vi "TrapezoidalMotionProfile.vi"(8 "dt":u32=20, 11 "Config":T1={"Distance"=200.0, "MaxVelocity"=100.0, "MaxAccel"=75.0, "InitialVelocity"=0.0, "FinalVelocity"=0.0}) -> (0 "dt":u32=20, 3 "Profile":cluster{"Pos":dbl, "Vel":dbl, "Accel":dbl}[](array[cluster]))   [LabVIEW 2016]
panel:
  out "Graph":dbl[][](graph)=[[0.0, 0.015000000000000001, 0.060000000000000005, 0.135, 0.24000000000000002, 0.37500000000000006, 0.54, 0.7350000000000001, 0.9600000000000001, 1.2149999999999999, 1.5000000000000002, 1.815, 2.16, 2.535, 2.9400000000000004, 3.375, 3.8400000000000003, 4.335000000000001, 4.859999999999999, 5.415, 6.000000000000001, 6.614999999999999, 7.26, 7.9350000000000005, 8.64, 9.375, 10.14, 10.935, 11.760000000000002, 12.614999999999998, 13.5, 14.415000000000001, 15.360000000000001, 16.335, 17.340000000000003, 18.375000000000004, 19.439999999999998, 20.535, 21.66, 22.815, 24.000000000000004, 25.215000000000003, 26.459999999999997, 27.734999999999996, 29.04, 30.375000000000004, 31.740000000000002, 33.135000000000005, 34.56, 36.015, 37.5, 39.015, 40.56, 42.135000000000005, 43.74, 45.37500000000001, 47.040000000000006, 48.735000000000014, 50.459999999999994, 52.214999999999996, 54.0, 55.815, 57.660000000000004, 59.535000000000004, 61.440000000000005, 63.37500000000001, 65.34, 67.33333333333334, 69.33333333333334, 71.33333333333334, 73.33333333333334, 75.33333333333333, 77.33333333333333, 79.33333333333333, 81.33333333333333, 83.33333333333333, 85.33333333333333, 87.33333333333334, 89.33333333333334, 91.33333333333334, 93.33333333333334, 95.33333333333334, 97.33333333333334, 99.33333333333334, 101.33333333333333, 103.33333333333333, 105.33333333333333, 107.33333333333333, 109.33333333333333, 111.33333333333334, 113.33333333333334, 115.33333333333334, 117.33333333333334, 119.33333333333334, 121.33333333333334, 123.33333333333334, 125.33333333333331, 127.33333333333333, 129.33333333333331, 131.33333333333331, 133.33333333333331, 135.31833333333338, 137.27333333333337, 139.19833333333338, 141.09333333333336, 142.95833333333337, 144.79333333333338, 146.59833333333336, 148.37333333333336, 150.11833333333337, 151.83333333333337, 153.51833333333337, 155.17333333333337, 156.79833333333337, 158.39333333333337, 159.95833333333337, 161.49333333333334, 162.99833333333333, 164.47333333333336, 165.91833333333335, 167.33333333333334, 168.71833333333336, 170.07333333333335, 171.39833333333334, 172.69333333333336, 173.95833333333334, 175.19333333333336, 176.39833333333337, 177.57333333333335, 178.71833333333336, 179.83333333333334, 180.91833333333335, 181.97333333333336, 182.99833333333336, 183.99333333333337, 184.95833333333334, 185.89333333333335, 186.79833333333335, 187.67333333333335, 188.51833333333335, 189.33333333333334, 190.11833333333334, 190.87333333333333, 191.59833333333333, 192.29333333333335, 192.95833333333334, 193.59333333333333, 194.19833333333335, 194.77333333333334, 195.31833333333333, 195.83333333333334, 196.31833333333333, 196.77333333333334, 197.19833333333335, 197.59333333333333, 197.95833333333334, 198.29333333333335, 198.59833333333333, 198.87333333333333, 199.11833333333334, 199.33333333333334, 199.51833333333335, 199.67333333333335, 199.79833333333335, 199.89333333333335, 199.95833333333334, 199.99333333333334, 199.99833333333333], [0.0, 1.5, 3.0, 4.5, 6.0, 7.5, 9.0, 10.500000000000002, 12.0, 13.5, 15.0, 16.5, 18.0, 19.5, 21.000000000000004, 22.5, 24.0, 25.500000000000004, 27.0, 28.5, 30.0, 31.5, 33.0, 34.5, 36.0, 37.5, 39.0, 40.5, 42.00000000000001, 43.5, 45.0, 46.5, 48.0, 49.5, 51.00000000000001, 52.50000000000001, 54.0, 55.5, 57.0, 58.5, 60.0, 61.50000000000001, 63.0, 64.5, 66.0, 67.5, 69.0, 70.5, 72.0, 73.5, 75.0, 76.5, 78.0, 79.5, 81.0, 82.5, 84.00000000000001, 85.50000000000001, 87.0, 88.5, 90.0, 91.5, 93.0, 94.5, 96.0, 97.5, 99.0, 100.0, 100.0, 100.0, 100.0, 100.0, 100.0, 100.0, 100.0, 100.0, 100.0, 100.0, 100.0, 100.0, 100.0, 100.0, 100.0, 100.0, 100.0, 100.0, 100.0, 100.0, 100.0, 100.0, 100.0, 100.0, 100.0, 100.0, 100.0, 100.0, 100.0, 100.0, 100.0, 100.0, 100.0, 98.5, 97.0, 95.5, 94.0, 92.5, 91.0, 89.49999999999999, 87.99999999999999, 86.49999999999999, 84.99999999999999, 83.49999999999999, 81.99999999999999, 80.49999999999999, 78.99999999999999, 77.49999999999997, 76.00000000000001, 74.50000000000001, 73.00000000000001, 71.5, 70.0, 68.5, 67.0, 65.5, 64.0, 62.5, 61.0, 59.5, 57.99999999999999, 56.49999999999999, 54.99999999999999, 53.49999999999999, 51.99999999999999, 50.499999999999986, 48.999999999999986, 47.499999999999986, 45.999999999999986, 44.499999999999986, 42.999999999999986, 41.49999999999998, 39.99999999999998, 38.500000000000014, 37.000000000000014, 35.500000000000014, 34.000000000000014, 32.5, 31.0, 29.5, 28.0, 26.5, 25.0, 23.5, 22.0, 20.5, 19.0, 17.5, 15.999999999999986, 14.499999999999986, 12.999999999999986, 11.499999999999986, 9.999999999999986, 8.499999999999986, 6.999999999999986, 5.499999999999986, 3.999999999999986, 2.499999999999986, 0.9999999999999716, -0.4999999999999858]]
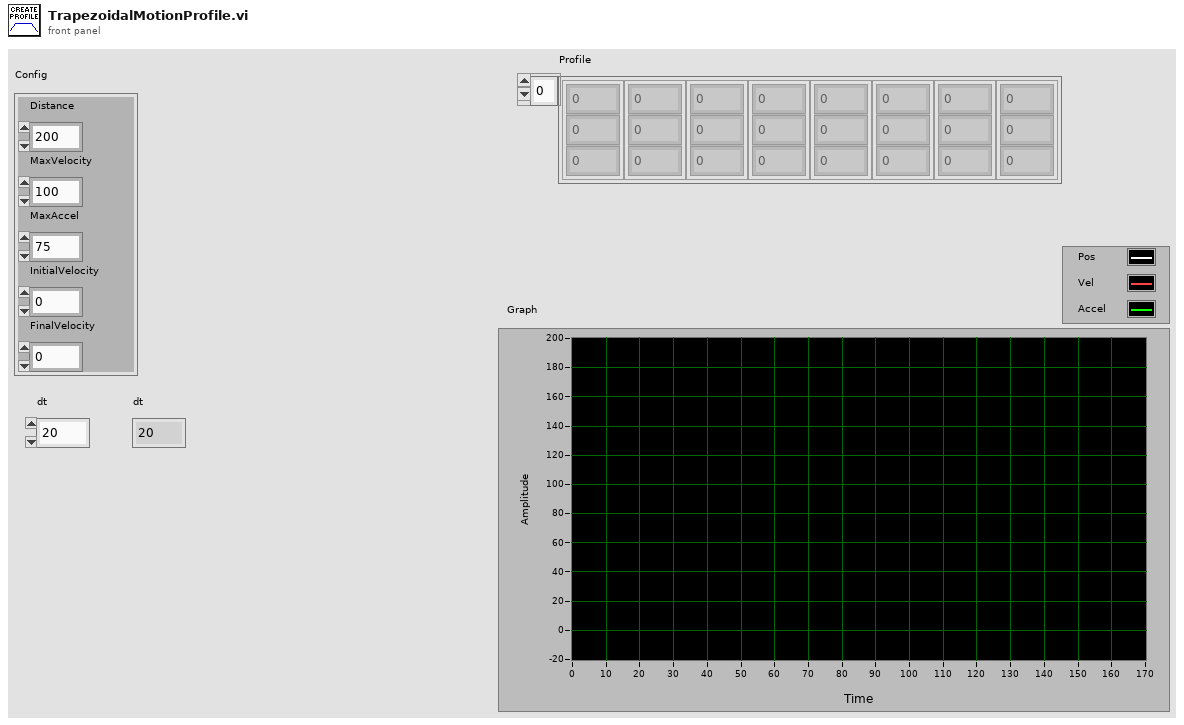
[diagram p1: front panel]
types:
  T1 = cluster{"Distance":dbl, "MaxVelocity":dbl, "MaxAccel":dbl, "InitialVelocity":dbl, "FinalVelocity":dbl}
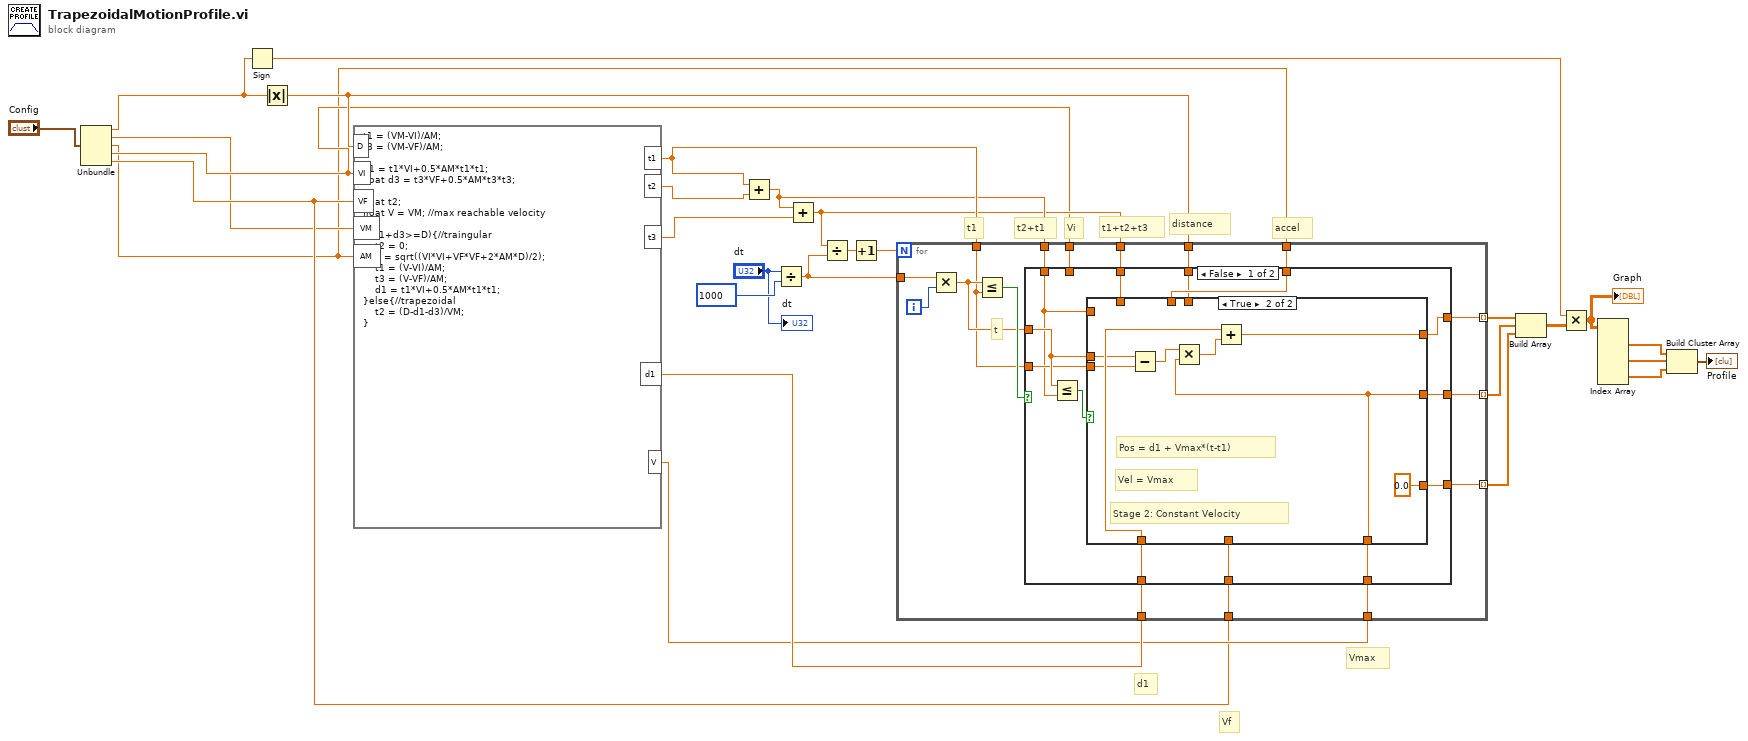
[diagram p0: block diagram]
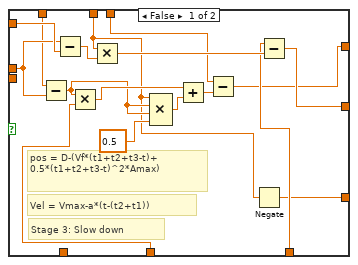
[diagram p2: hidden frame]
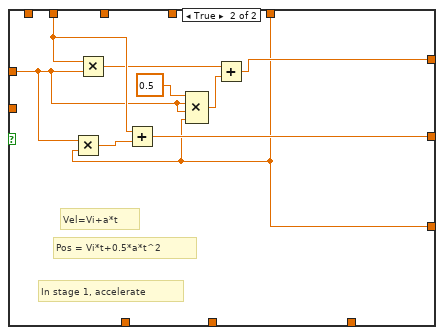
[diagram p3: hidden frame]
diagram:
  # "distance"
  # "Vf"
  # "t1+t2+t3"
  # "d1"
  # "Vmax"
  # "t1"
  # "t2+t1"
  # "Vi"
  # "accel"
  n1 = Unbundle("Config") -> ("Distance"=w5:dbl, "MaxVelocity"=w2:dbl, "MaxAccel"=w1:dbl, "InitialVelocity"=w4:dbl, "FinalVelocity"=w3:dbl)
  n2 = Sign(1:w5) -> (0:w12:dbl)
  n3 = Absolute Value(x=w5) -> (abs(x)=w14:dbl)
  n4 = formula code="t1 = (VM-VI)/AM;\nt3 = (VM-VF)/AM;\n\nd1 = t1*VI+0.5*AM*t1*t1;\nfloat d3 = t3*VF+0.5*AM*t3*t3;\n\nfloat t2;\nfloat V = VM; //max reachable velocity\n\nif(d1+d3>=D){//traingular\n    t2 = 0;\n    V = sqrt((VI*VI+VF*VF+2*AM*D)/2);\n    t1 = (V-VI)/AM;\n    t3 = (V-VF)/AM;\n    d1 = t1*VI+0.5*AM*t1*t1;\n}else{//trapezoidal\n    t2 = (D-d1-d3)/VM;\n}"("VI"=w4, "VF"=w3, "D"=w14, "VM"=w2, "AM"=w1) -> ("t1"=w23:dbl, "t3"=w28:dbl, "d1"=w21:dbl, "t2"=w29:dbl, "V"=w16:dbl)
  n5 = Add(x=w23, y=w29) -> (x+y=w22:dbl)
  n6 = Divide(x="dt", y=u32 1000) -> (x/y=w24:dbl)
  n7 = Add(x=w22, y=w28) -> (x+y=w18:dbl)
  n8 = Divide(x=w18, y=w24) -> (x/y=w26:dbl)
  n9 = Increment(x=w26) -> (x+1=w25:dbl)
  n10 = for {
    N: w25 -> [_]
    tunnel: w24 -> [w44]
    tunnel: w23 -> [w34]
    tunnel: w4 -> [w42]
    tunnel: w1 -> [w41]
    tunnel: [w40] -> w19 mode=indexing
    tunnel: [w39] -> w20 mode=indexing
    tunnel: w22 -> [w38]
    tunnel: w16 -> [w36]
    tunnel: w21 -> [w35]
    tunnel: w18 -> [w33]
    tunnel: w3 -> [w32]
    tunnel: w14 -> [w31]
    tunnel: [w30] -> w15 mode=indexing
    i -> [w45]
    # "t"
    n11 = Multiply(x=w44, y=w45) -> (x*y=w37:dbl)
    n12 = Less Or Equal?(x=w37, y=w34) -> (x <= y?=w43:bool)
    n13 = case shown="False" w43 {
      tunnel: w42 -> [_ w90]
      tunnel: w41 -> [w50 w84]
      tunnel: w37 -> [w54 w87]
      tunnel: [w57 w91] -> w40
      tunnel: [w52 w85] -> w39
      tunnel: w38 -> [w51 _]
      tunnel: w36 -> [w56 _]
      tunnel: w35 -> [w55 _]
      tunnel: w34 -> [w53 _]
      tunnel: w33 -> [w49 _]
      tunnel: w32 -> [w48 _]
      tunnel: w31 -> [w47 _]
      tunnel: [w46 w84] -> w30
      frame False {
        n14 = Less Or Equal?(x=w54, y=w51) -> (x <= y?=w58:bool)
        n15 = case shown="True" w58 {
          tunnel: [w71 w80] -> w57
          tunnel: w56 -> [w72 w80]
          tunnel: w55 -> [_ w83]
          tunnel: w54 -> [w70 w82]
          tunnel: w53 -> [_ w81]
          tunnel: [w61 w77] -> w52
          tunnel: w51 -> [w75 _]
          tunnel: w50 -> [w59 _]
          tunnel: w49 -> [w69 _]
          tunnel: w48 -> [w68 _]
          tunnel: w47 -> [w62 _]
          tunnel: [w60 0.0] -> w46
          frame False {
            # "pos = D-(Vf*(t1+t2+t3-t)+\n0.5*(t1+t2+t3-t)^2*Amax)"
            # "Vel = Vmax-a*(t-(t2+t1))"
            # "Stage 3: Slow down"
            n16 = Subtract(x=w69, y=w70) -> (x-y=w65:dbl)
            n17 = Subtract(x=w70, y=w75) -> (x-y=w74:dbl)
            n18 = Multiply(x=w65, y=w68) -> (x*y=w67:dbl)
            n19 = Multiply(x=w59, y=w74) -> (x*y=w73:dbl)
            n20 = Compound Arithmetic op=MULTIPLY(w59, w65, w65, 0.5 ("value")) -> (w64:dbl)
            n21 = Add(x=w67, y=w64) -> (x+y=w63:dbl)
            n22 = Subtract(x=w62, y=w63) -> (x-y=w61:dbl)
            n23 = Negate(x=w59) -> (-x=w60:dbl)
            n24 = Subtract(x=w72, y=w73) -> (x-y=w71:dbl)
          }
          frame True {
            # "Pos = d1 + Vmax*(t-t1)"
            # "Vel = Vmax"
            # "Stage 2: Constant Velocity"
            n25 = Subtract(x=w82, y=w81) -> (x-y=w79:dbl)
            n26 = Multiply(x=w79, y=w80) -> (x*y=w78:dbl)
            n27 = Add(x=w83, y=w78) -> (x+y=w77:dbl)
          }
        }
      }
      frame True {
        # "Vel=Vi+a*t"
        # "Pos = Vi*t+0.5*a*t^2"
        # "In stage 1, accelerate"
        n28 = Multiply(x=w87, y=w84) -> (x*y=w92:dbl)
        n29 = Multiply(x=w90, y=w87) -> (x*y=w89:dbl)
        n30 = Add(x=w90, y=w92) -> (x+y=w91:dbl)
        n31 = Compound Arithmetic op=MULTIPLY(0.5 ("t2"), w87, w87, w84) -> (w86:dbl)
        n32 = Add(x=w89, y=w86) -> (x+y=w85:dbl)
      }
    }
  }
  n33 = Build Array(w20, w19, w15) -> (w13:dbl[][])
  n34 = Multiply(x=w12, y=w13) -> (x*y=w11:dbl[][])
  "Graph" <- w11
  n35 = Index Array(array=w11) -> (element #1=w10:dbl[], element #2=w9:dbl[], element #3=w8:dbl[])  [unwired: 6 in]
  n36 = Build Cluster Array(w10, w9, w8) -> (→"Profile":cluster{dbl, dbl, dbl}[])
  "dt" <- "dt"
